vi "LJM logger prompt new program config.vi"(10 "Program Configs In":T2={"Data File Prefix"="", "Scan Rate (Hz)"=0.0, "Graph History"=0, "# Channels"=0, "Disable Scaling"=FALSE, "Max File Size (Bytes)"=0, "Channel Setup 2"={"Name"=["AIN0", "AIN1", "AIN2", "AIN3", "AIN4", "AIN5", "AIN6", "AIN7", "AIN8", "AIN9", "AIN10", "AIN11", "AIN12", "AIN13", "AIN14", "AIN15"], "", "Scaling Equation"=["y=a", "y=b", "y=c", "y=d", "y=e", "y=f", "y=g", "y=h", "y=i", "y=j", "y=k", "y=l", "y=m", "y=n", "y=o", "y=p"], "", "Graph?"=[TRUE, TRUE, TRUE, TRUE, FALSE, FALSE, FALSE, FALSE, FALSE, FALSE, FALSE, FALSE, FALSE, FALSE, FALSE, FALSE]}, "Interval (ms)"=0, "Write To File"=FALSE, "Log Every n Scans"=0}, 11 "Working Directory In":path) -> (0 "error out":errorcluster, 1 "New Program Config Name":string, 2 "Program Configs Out":T2={"Data File Prefix"="", "Scan Rate (Hz)"=0.0, "Graph History"=0, "# Channels"=0, "Disable Scaling"=FALSE, "Max File Size (Bytes)"=0, "Channel Setup 2"={"Name"=["AIN0", "AIN1", "AIN2", "AIN3", "AIN4", "AIN5", "AIN6", "AIN7", "AIN8", "AIN9", "AIN10", "AIN11", "AIN12", "AIN13", "AIN14", "AIN15"], "", "Scaling Equation"=["y=a", "y=b", "y=c", "y=d", "y=e", "y=f", "y=g", "y=h", "y=i", "y=j", "y=k", "y=l", "y=m", "y=n", "y=o", "y=p"], "", "Graph?"=[TRUE, TRUE, TRUE, TRUE, FALSE, FALSE, FALSE, FALSE, FALSE, FALSE, FALSE, FALSE, FALSE, FALSE, FALSE, FALSE]}, "Interval (ms)"=0, "Write To File"=FALSE, "Log Every n Scans"=0})   [LabVIEW 2026]
uses:
  Common Logger Controls/Channel Setup.ctl
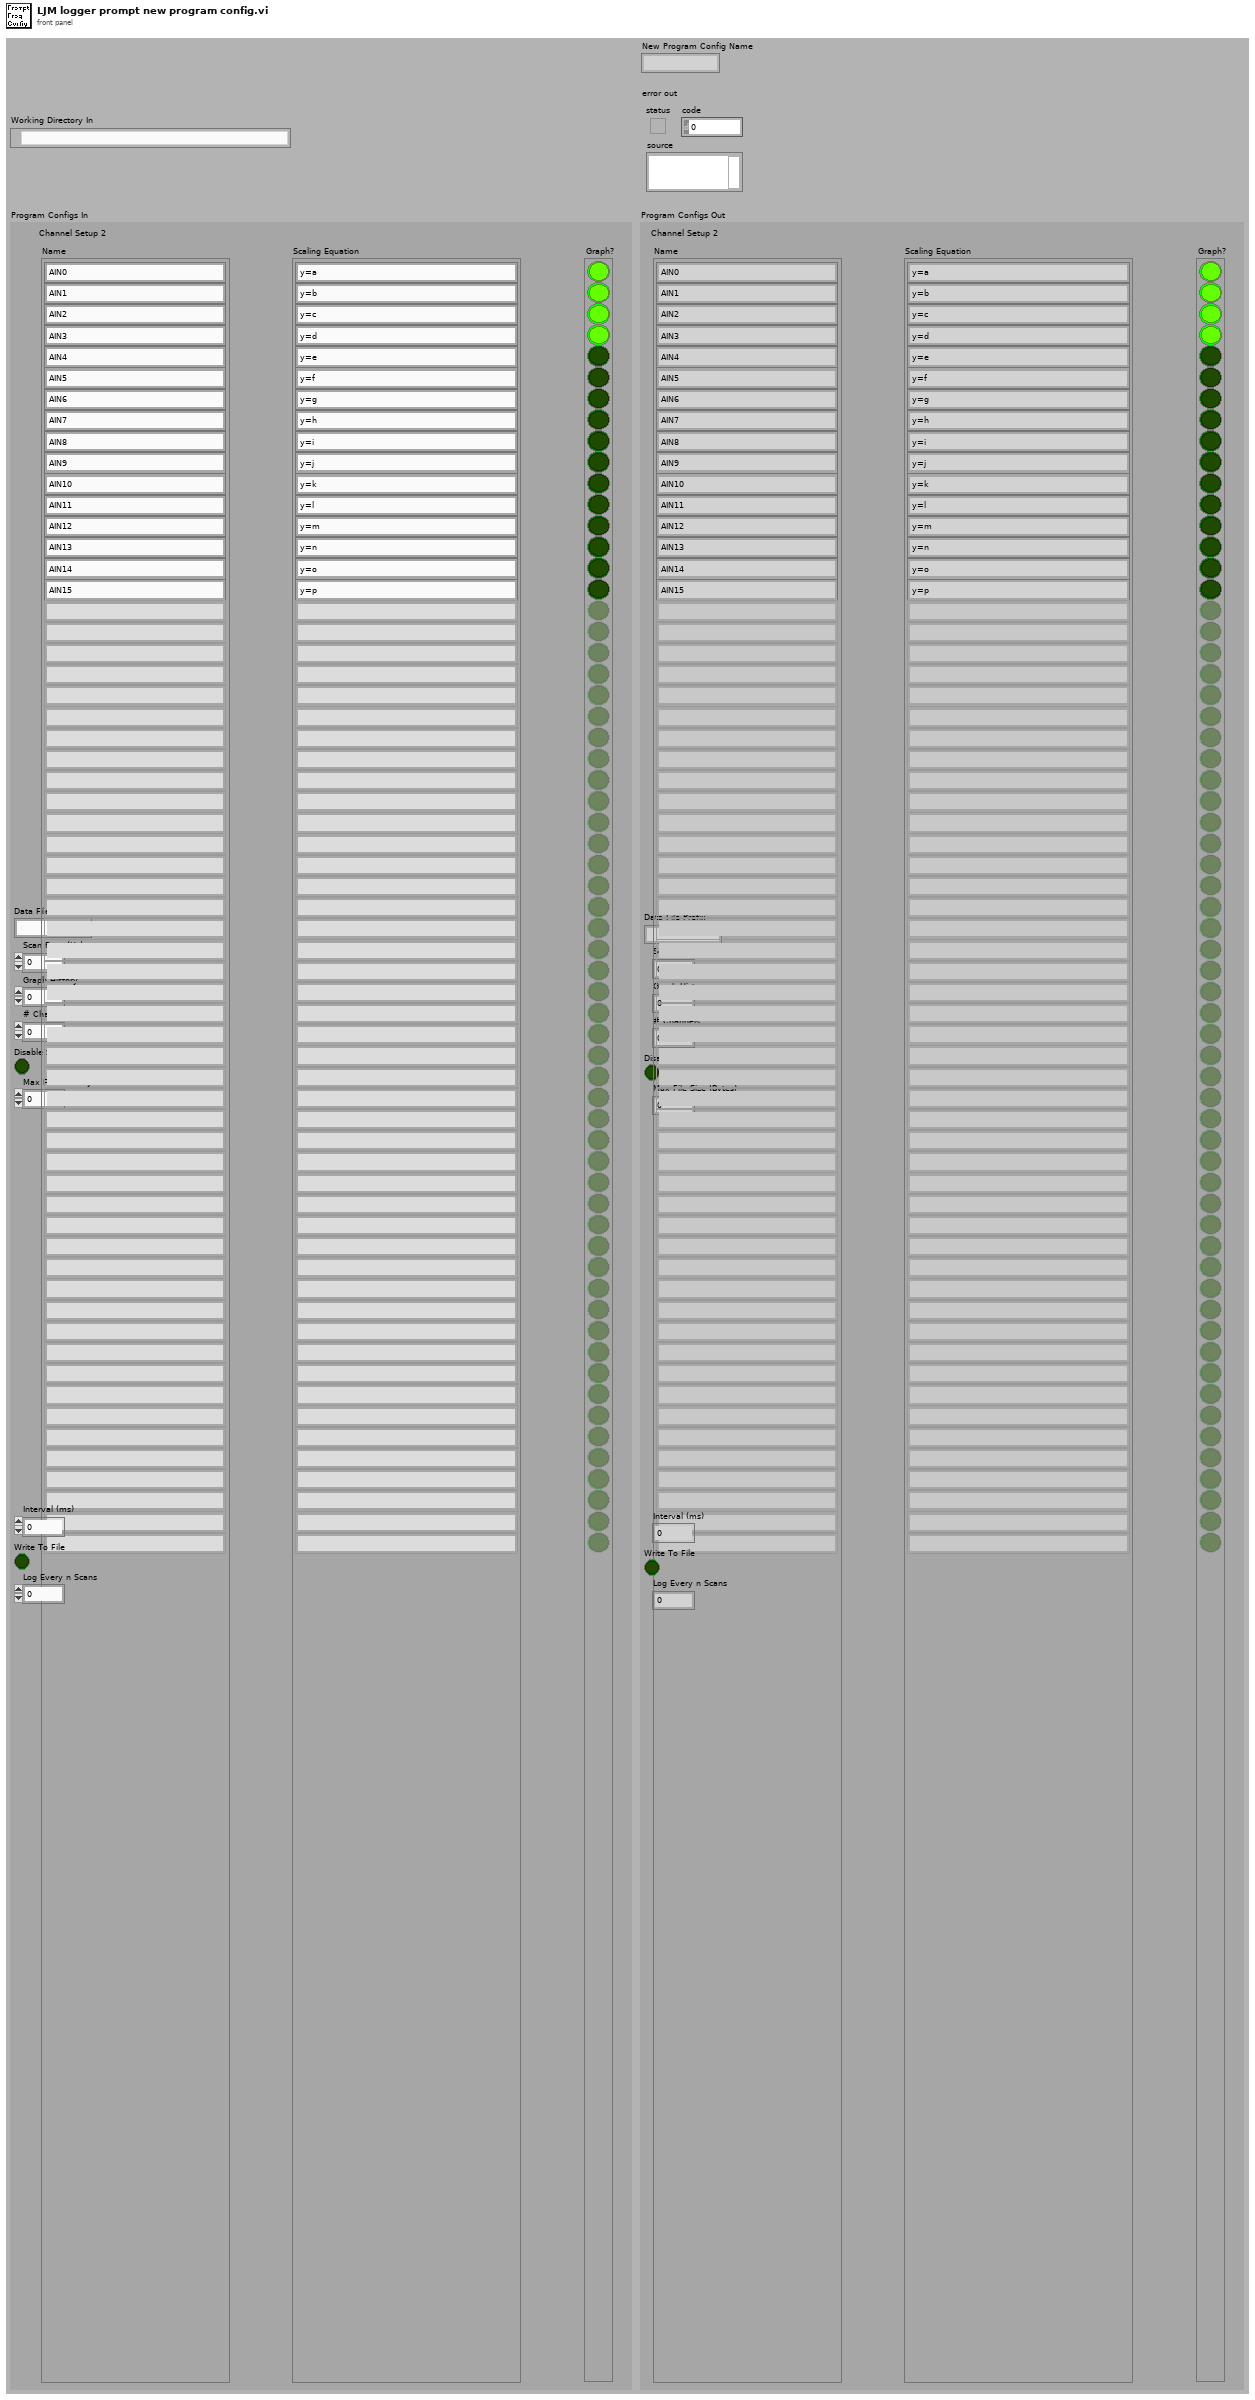
[diagram p1: front panel]
types:
  T1 = typedef "Channel Setup.ctl" = cluster{"Name":string[], string, "Scaling Equation":string[], string, "Graph?":bool[]}
  T2 = cluster{"Data File Prefix":string, "Scan Rate (Hz)":dbl, "Graph History":i32, "# Channels":i32, "Disable Scaling":bool, "Max File Size (Bytes)":i32, "Channel Setup 2":T1, "Interval (ms)":u32, "Write To File":bool, "Log Every n Scans":i32}
  T3 = enum32{"existing file", "new file", "new or existing file", "existing dir", "new dir", "new or existing dir", "existing file (use LLBs)", "new file (use LLBs)", "new or existing file (use LLBs)", "new or existing file or directory (use LLBs)"}
  T4 = typedef "Program Config Cluster.ctl" = cluster{"Data File Prefix":string, "Scan Rate (Hz)":dbl, "Graph History":i32, "# Channels":i32, "Disable Scaling":bool, "Max File Size (Bytes)":i32, "Channel Setup":T1, "Interval (ms)":u32, "Write To File":bool, "Log Every n Scans":i32}
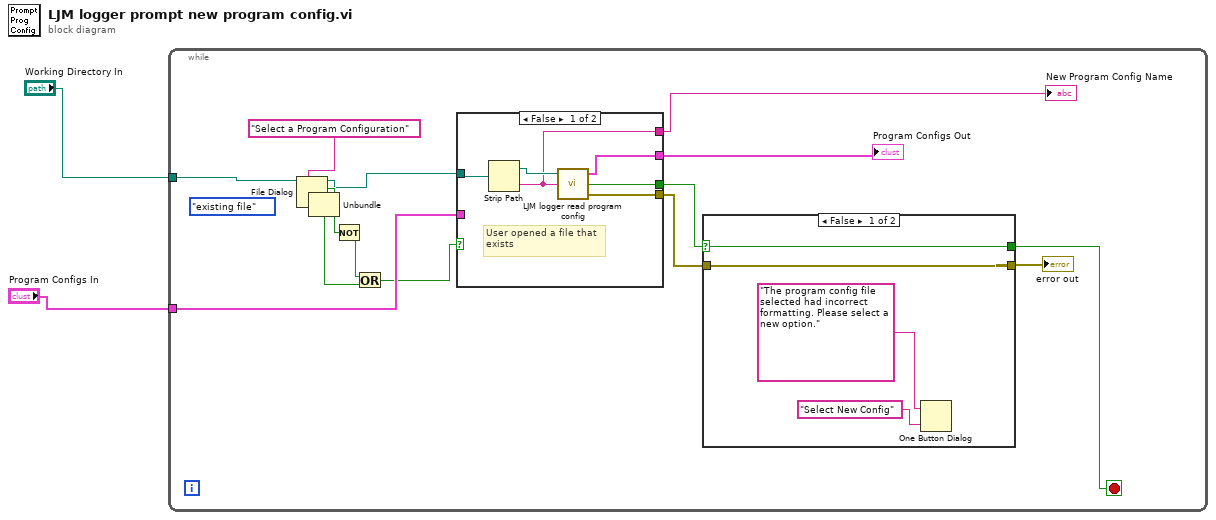
[diagram p0: block diagram]
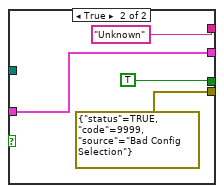
[diagram p2: hidden frame]
diagram:
  n1 = while {
    tunnel: "Working Directory In" -> [w16]
    tunnel: "Program Configs In" -> [w12]
    stop <- w5 stop-if-true
    (unwired) T3."existing file" ("select mode (2)")
    n2 = File Dialog(7:"Select a Program Configuration" ("Substring"), 11:w16) -> (0:w3:errorcluster, 1:w8:bool, 2:w9:bool, 3:w7:path)  [unwired: 5 in]
    n3 = Unbundle(w3) -> ()  [unwired: 3 out]
    n4 = Not(x=w9) -> (.not. x?=w11:bool)
    n5 = Or(x=w11, y=w8) -> (x .or. y?=w10:bool)
    n6 = case shown="False" w10 {
      tunnel: [w23 w25] -> w4
      tunnel: [w22 errorcluster {"status"=TRUE, "code"=9999, "source"="Bad Config Selection"} ("error out")] -> w14
      tunnel: w7 -> [w18 _]
      tunnel: [w21 TRUE ("Good Experiment Config")] -> w13
      tunnel: w12 -> [_ w25]
      tunnel: [w19 "Unknown" ("name")] -> w6
      frame False {
        # "User opened a file that\nexists"
        n7 = Strip Path(path=w18) -> (stripped path=w20:path, name=w19:string)
        n8 = call "LJM logger read program config.vi"("filename"=w19, "Working Directory"=w20) -> ("error out"=w22:errorcluster, "Good Program Config"=w21:bool, "Program Configs Out"=w23:T4)  [unwired: 1 in]
      }
      frame True {
      }
    }
    "New Program Config Name" <- w6
    "Program Configs Out" <- w4
    n9 = case shown="False" w13 {
      selector: w13 -> [w28 w32]
      tunnel: w14 -> [w31 w33]
      tunnel: [w31 w33] -> w17
      tunnel: [w28 w32] -> w5
      frame False {
        n10 = One Button Dialog(message="The program config file selected had incorrect formatting. Please select a new option.", button name ("OK")="Select New Config" ("T button name (\"OK\")")) -> ()  [unwired: 1 out]
      }
      frame True {
      }
    }
    "error out" <- w17
  }
